vi "Startup.vi"(6 "LabVIEW Web Service":refnum<class "Web Service.lvclass">) -> ()   [LabVIEW 2017]
uses:
  <vilib>/wsapi/Web Service.lvclass
  Controller/gController.lvclass
  C:/Program Files (x86)/National Instruments/LabVIEW 2017/vi.lib/ActorFramework/Actor/Actor.lvclass
  <vilib>/ActorFramework/Actor/Actor.lvclass
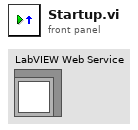
[diagram p1: front panel]
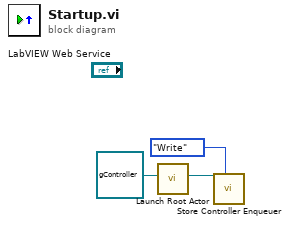
[diagram p0: block diagram]
diagram:
  n1 = call <vilib>:"Launch Root Actor.vi"("Actor"=refnum<class "gController.lvclass"> refnum ("gController.lvclass")) -> ("Actor's Enqueuer"=w2:refnum<class "Message Enqueuer.lvclass">)  [unwired: 9 in, 1 out]
  n2 = call "Store Controller Enqueuer.vi"("State"=enum16{"Write", "Read"}."Write", "Controller Enqueuer In"=w2) -> ()  [unwired: 9 in, 1 out]
